vi "IsGreaterOrEqual.vi"(1 "B":refnum<vi>, 2 "A":refnum<vi>) -> (0 "A greater or equal B ?":bool)   [LabVIEW 2013]
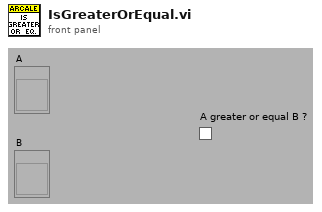
[diagram p1: front panel]
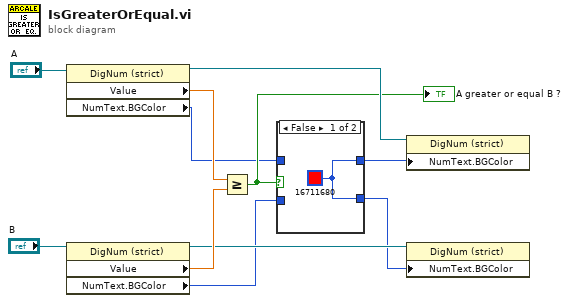
[diagram p0: block diagram]
diagram:
  n1 = property class="DigNum (strict)"(reference="A") -> (reference out=w7:refnum<vi>, "Value"=w9:dbl, "NumText.BGColor"=w2:u32)  [unwired: 1 in, 1 out]
  n2 = property class="DigNum (strict)"(reference="B") -> (reference out=w6:refnum<vi>, "Value"=w8:dbl, "NumText.BGColor"=w1:u32)  [unwired: 1 in, 1 out]
  n3 = Greater Or Equal?(x=w9, y=w8) -> (x >= y?=w3:bool)
  "A greater or equal B ?" <- w3
  n4 = case shown="False" w3 {
    tunnel: [w12 w13] -> w5
    tunnel: [w12 w14] -> w4
    tunnel: w2 -> [_ w14]
    tunnel: w1 -> [_ w13]
    frame False {
      w12 = u32 16711680
    }
    frame True {
    }
  }
  n5 = property class="DigNum (strict)"(reference=w7, "NumText.BGColor"=w4) -> ()  [unwired: 1 in, 2 out]
  n6 = property class="DigNum (strict)"(reference=w6, "NumText.BGColor"=w5) -> ()  [unwired: 1 in, 2 out]
